vi "frontEnd.vi"(8 "error in (no error)":errorcluster, 11 "ScriptEditorV2 in":refnum<class "ScriptEditorV2.lvclass">) -> (0 "error out":errorcluster, 3 "ScriptEditorV2 out":refnum<class "ScriptEditorV2.lvclass">)   [LabVIEW 2011, in "Views.lvlib" / "ScriptEditor.lvlib" / "ScriptEditorV2.lvclass"]
uses:
  ScriptEditorV2.lvclass
  ScriptEditorV2.lvclass/ScriptEditorV2.ctl
  ScriptEdEvents/ScriptEdEvents.lvclass
  Tools/DatabaseHelpers.lvlib
panel:
  in  "Delete Event":bool
  in  "highlightChannel":bool
  in  "open":bool
  in  "saveAs":bool
  in  "save":bool
  in  "Script Information":string
  out "Multicolumn Listbox":i32[](listbox)
  # "Open"
  # "save"
  # "saveAs"
  # "Highlight"
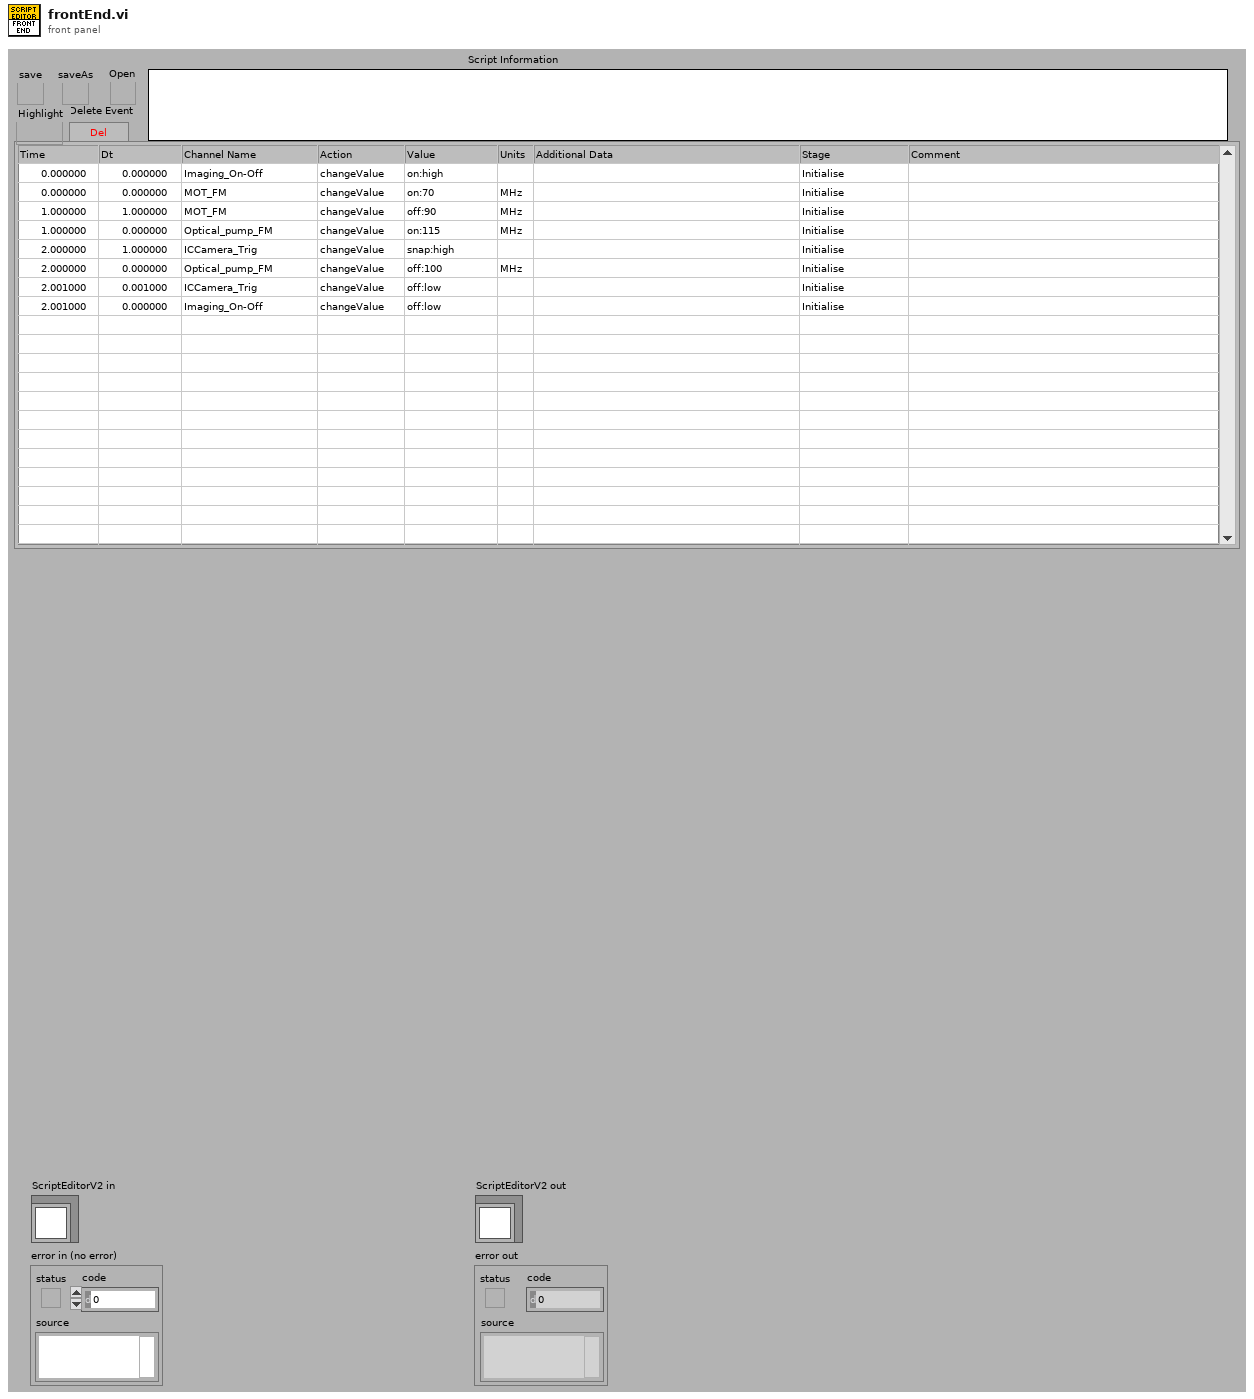
[diagram p1: front panel]
types:
  T1 = typedef "LVPoint32TypeDef.ctl" = cluster{"Horizontal":i32, "Vertical":i32}
  T2 = typedef "LVRowAndColumnTypeDef.ctl" = cluster{"Row":i32, "Column":i32}
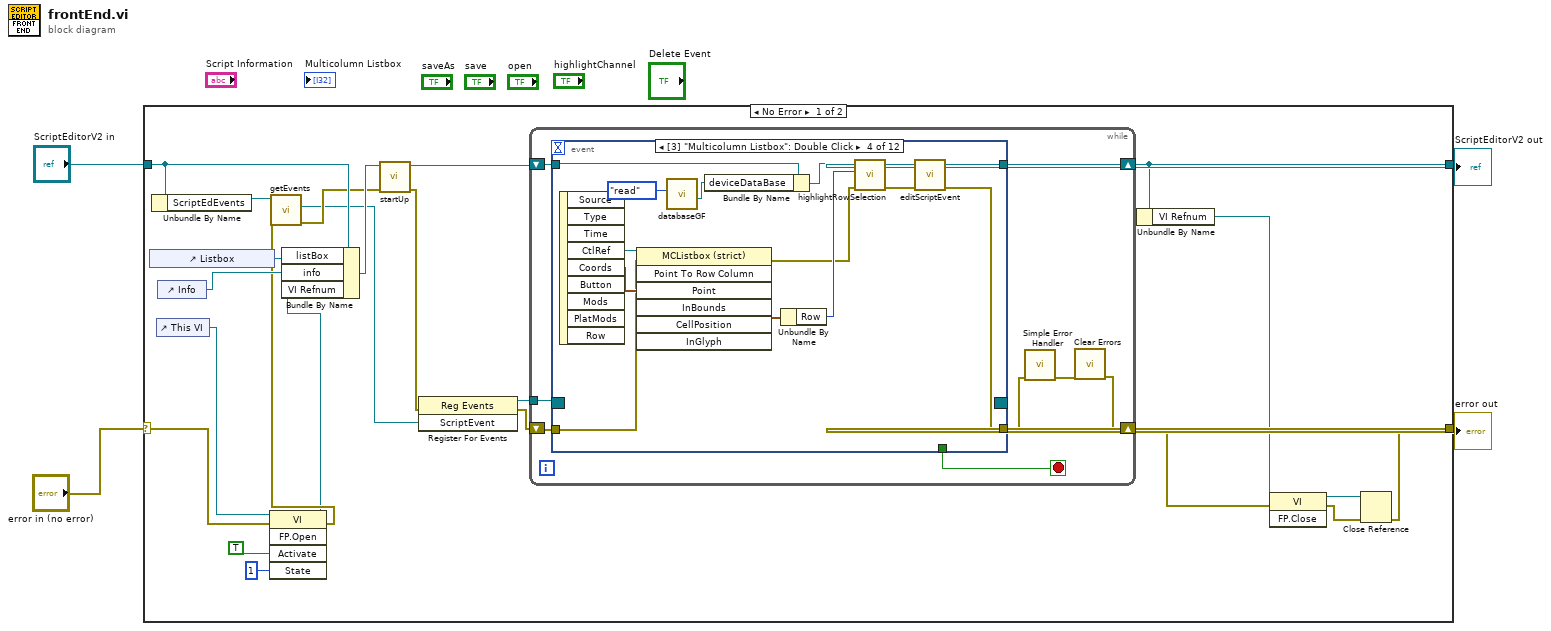
[diagram p0: block diagram]
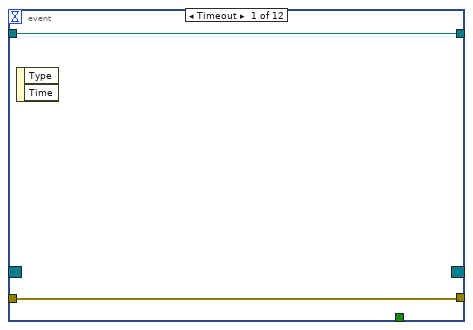
[diagram p2: hidden frame]
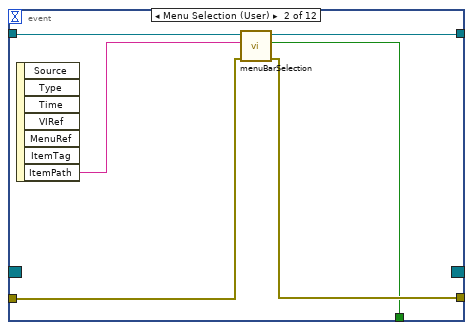
[diagram p3: hidden frame]
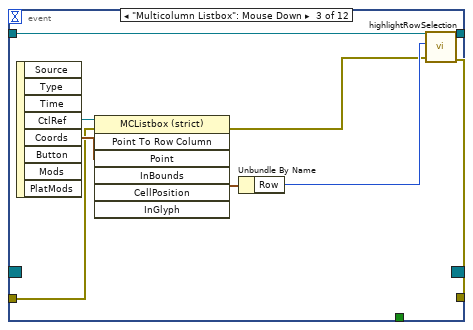
[diagram p4: hidden frame]
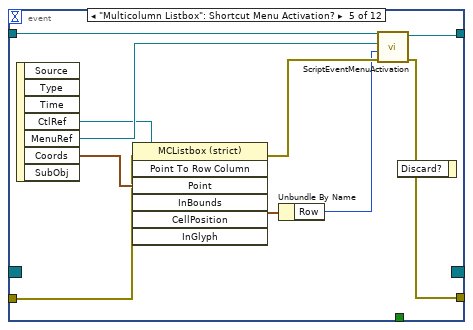
[diagram p5: hidden frame]
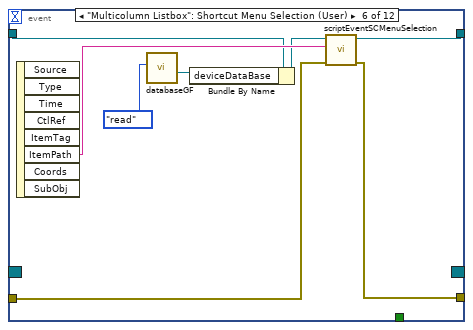
[diagram p6: hidden frame]
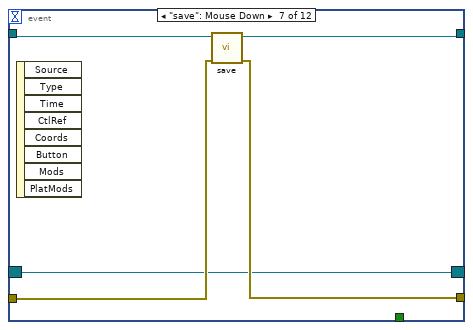
[diagram p7: hidden frame]
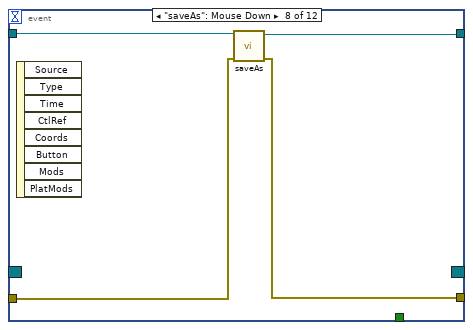
[diagram p8: hidden frame]
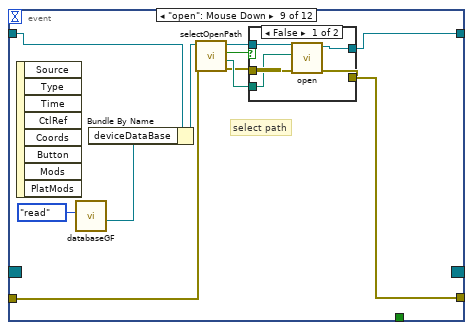
[diagram p9: hidden frame]
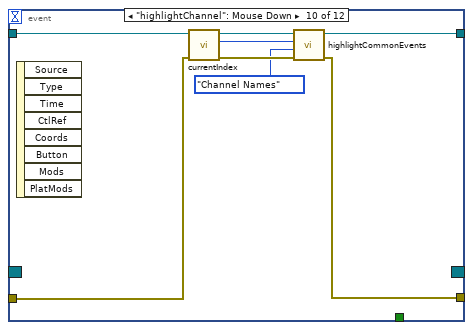
[diagram p11: hidden frame]
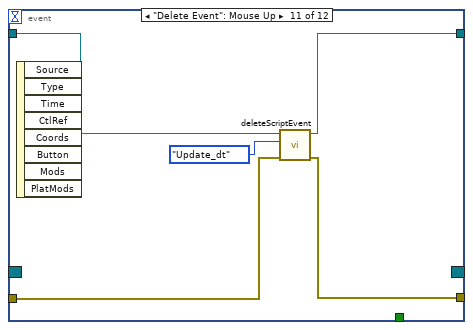
[diagram p12: hidden frame]
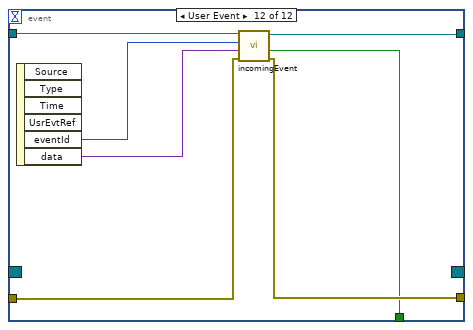
[diagram p13: hidden frame]
diagram:
  n1 = case shown="No Error" "error in (no error)" {
    selector: "error in (no error)" -> [w13 w133]
    tunnel: [w5 w133] -> w3
    tunnel: [w10 w132] -> w1
    tunnel: "ScriptEditorV2 in" -> [w24 w132]
    frame No Error {
      n2 = control-ref of="Listbox"() -> (w17:refnum<vi>)
      n3 = Unbundle By Name(w24) -> ("ScriptEdEvents"=w23:refnum<class "ScriptEdEvents.lvclass">)
      n4 = control-ref of="This VI"() -> (w14:refnum<vi>)
      n5 = control-ref of="Info"() -> (w26:refnum<vi>)
      n6 = invoke class="VI" method="FP.Open"(reference=w14, error in=w13, "Activate"=TRUE, "State"=1) -> (reference out=w11:refnum<vi>, error out=w12:errorcluster)  [unwired: 1 in, 3 out]
      n7 = call-dynamic "getEvents.vi"("error in (no error)"=w12, "ScriptEdEvents in"=w23) -> ("error out"=w21:errorcluster, "ScriptEvent"=w20:refnum<user-event>)  [unwired: 6 in, 2 out]
      n8 = Bundle By Name(cluster=w24, "listBox"=w17, "info"=w26, "VI Refnum"=w11) -> (w25:refnum<class "ScriptEditorV2.lvclass">)
      n9 = call "startUp.vi"("error in (no error)"=w21, "ScriptEditorV2 in"=w25) -> ("error out"=w18:errorcluster, "ScriptEditorV2 out"=w27:refnum<class "ScriptEditorV2.lvclass">)  [unwired: 8 in]
      n10 = register-events(error in=w18, w20) -> (reference out=w22:refnum<event-registration>, error out=w19:errorcluster)  [unwired: 1 in]
      n11 = while {
        shift-right: [w35] -> w10
        shift-left: w27 -> [w31]
        shift-right: [w28] -> w8
        shift-left: w19 -> [w34]
        tunnel: w22 -> [w32]
        stop <- w33 stop-if-true
        n12 = event shown="[3] \"Multicolumn Listbox\": Double Click" {
          selector: w32 -> [_ _ _ _ _ _ w85 _ _ _ _ _]
          dyn-events: [_ _ _ _ _ _ w85 _ _ _ _ _] -> _
          timeout: _ -> [_ _ _ _ _ _ _ _ _ _ _ _]
          tunnel: w31 -> [w37 w43 w45 w54 w76 w79 w89 w93 w96 w115 w121 w131]
          tunnel: [w37 w42 w48 w58 w75 w84 w88 w92 w100 w114 w120 w130] -> w35
          tunnel: [w36 w40 w47 w57 w74 w82 w86 w90 w99 w112 w122 w128] -> w30
          tunnel: w34 -> [w36 w41 w50 w63 w70 w83 w87 w91 w98 w113 w123 w129]
          tunnel: [_ w39 _ _ _ _ _ _ _ _ _ w125] -> w33
          event Timeout {
            n13 = event-data() -> ()  [unwired: 1 in, 2 out]
          }
          event Menu Selection (User) {
            n14 = event-data() -> ("ItemPath"=w38:string)  [unwired: 1 in, 6 out]
            n15 = call "menuBarSelection.vi"("error in (no error)"=w41, "itemPath"=w38, "ScriptEditorV2 in"=w43) -> ("error out"=w40:errorcluster, "close"=w39:bool, "ScriptEditorV2 out"=w42:refnum<class "ScriptEditorV2.lvclass">)  [unwired: 6 in]
          }
          event "Multicolumn Listbox": Mouse Down {
            n16 = event-data() -> ("CtlRef"=w52:refnum<vi>, "Coords"=w51:T1)  [unwired: 1 in, 6 out]
            n17 = invoke class="MCListbox (strict)" method="Point To Row Column"(reference=w52, error in=w50, "Point"=w51) -> (error out=w44:errorcluster, "CellPosition"=w49:T2)  [unwired: 4 in, 5 out]
            n18 = Unbundle By Name(w49) -> ("Row"=w46:i32)
            n19 = call "highlightRowSelection.vi"("error in (no error)"=w44, "rowIndex"=w46, "ScriptEditorV2 in"=w45) -> ("error out"=w47:errorcluster, "ScriptEditorV2 out"=w48:refnum<class "ScriptEditorV2.lvclass">)  [unwired: 7 in]
          }
          event "Multicolumn Listbox": Double Click {
            n20 = event-data() -> ("CtlRef"=w65:refnum<vi>, "Coords"=w64:T1)  [unwired: 1 in, 7 out]
            n21 = invoke class="MCListbox (strict)" method="Point To Row Column"(reference=w65, error in=w63, "Point"=w64) -> (error out=w61:errorcluster, "CellPosition"=w66:T2)  [unwired: 4 in, 5 out]
            n22 = call "databaseGF.vi"("Enum"=enum16{"write", "read"}."read") -> ("deviceDataBase out"=w55:refnum<class "deviceDataBase.lvclass">)  [unwired: 10 in]
            n23 = Bundle By Name(cluster=w54, "deviceDataBase"=w55) -> (w53:refnum<class "ScriptEditorV2.lvclass">)
            n24 = Unbundle By Name(w66) -> ("Row"=w62:i32)
            n25 = call "highlightRowSelection.vi"("error in (no error)"=w61, "rowIndex"=w62, "ScriptEditorV2 in"=w53) -> ("error out"=w59:errorcluster, "ScriptEditorV2 out"=w60:refnum<class "ScriptEditorV2.lvclass">)  [unwired: 7 in]
            n26 = call "editScriptEvent.vi"("error in (no error)"=w59, "ScriptEditorV2 in"=w60) -> ("error out"=w57:errorcluster, "ScriptEditorV2 out"=w58:refnum<class "ScriptEditorV2.lvclass">)  [unwired: 8 in]
          }
          event "Multicolumn Listbox": Shortcut Menu Activation? {
            n27 = event-data() -> ("CtlRef"=w72:refnum<vi>, "MenuRef"=w73:refnum<k9>, "Coords"=w71:T1)  [unwired: 1 in, 4 out]
            n28 = invoke class="MCListbox (strict)" method="Point To Row Column"(reference=w72, error in=w70, "Point"=w71) -> (error out=w68:errorcluster, "CellPosition"=w69:T2)  [unwired: 4 in, 5 out]
            n29 = Unbundle By Name(w69) -> ("Row"=w67:i32)
            n30 = call "ScriptEventMenuActivation.vi"("error in (no error)"=w68, "rowIndex"=w67, "MenuRef"=w73, "ScriptEditorV2 in"=w76) -> ("error out"=w74:errorcluster, "ScriptEditorV2 out"=w75:refnum<class "ScriptEditorV2.lvclass">)  [unwired: 6 in]
            n31 = event-data() -> ()  [unwired: 2 in, 1 out]
          }
          event "Multicolumn Listbox": Shortcut Menu Selection (User) {
            n32 = event-data() -> ("ItemPath"=w81:string)  [unwired: 1 in, 7 out]
            n33 = call "databaseGF.vi"("Enum"=enum16{"write", "read"}."read") -> ("deviceDataBase out"=w77:refnum<class "deviceDataBase.lvclass">)  [unwired: 10 in]
            n34 = Bundle By Name(cluster=w79, "deviceDataBase"=w77) -> (w78:refnum<class "ScriptEditorV2.lvclass">)
            n35 = call "scriptEventSCMenuSelection.vi"("error in (no error)"=w83, "path"=w81, "ScriptEditorV2 in"=w78) -> ("error out"=w82:errorcluster, "ScriptEditorV2 out"=w84:refnum<class "ScriptEditorV2.lvclass">)  [unwired: 7 in]
          }
          event "save": Mouse Down {
            n36 = event-data() -> ()  [unwired: 1 in, 8 out]
            n37 = call "save.vi"("error in (no error)"=w87, "ScriptEditorV2 in"=w89) -> ("error out"=w86:errorcluster, "ScriptEditorV2 out"=w88:refnum<class "ScriptEditorV2.lvclass">)  [unwired: 8 in]
          }
          event "saveAs": Mouse Down {
            n38 = event-data() -> ()  [unwired: 1 in, 8 out]
            n39 = call "saveAs.vi"("error in (no error)"=w91, "ScriptEditorV2 in"=w93) -> ("error out"=w90:errorcluster, "ScriptEditorV2 out"=w92:refnum<class "ScriptEditorV2.lvclass">)  [unwired: 8 in]
          }
          event "open": Mouse Down {
            # "select path"
            n40 = event-data() -> ()  [unwired: 1 in, 8 out]
            n41 = call "databaseGF.vi"("Enum"=enum16{"write", "read"}."read") -> ("deviceDataBase out"=w94:refnum<class "deviceDataBase.lvclass">)  [unwired: 10 in]
            n42 = Bundle By Name(cluster=w96, "deviceDataBase"=w94) -> (w95:refnum<class "ScriptEditorV2.lvclass">)
            n43 = call "selectOpenPath.vi"("error in (no error)"=w98, "ScriptEditorV2 in"=w95) -> ("error out"=w101:errorcluster, "selected path"=w103:path, "notSelected?"=w102:bool, "ScriptEditorV2 out"=w104:refnum<class "ScriptEditorV2.lvclass">)  [unwired: 6 in]
            n44 = case shown="False" w102 {
              tunnel: [w109 w111] -> w100
              tunnel: w101 -> [w108 w110]
              tunnel: [w107 w110] -> w99
              tunnel: w104 -> [w106 w111]
              tunnel: w103 -> [w105 _]
              frame False {
                n45 = call "open.vi"("error in (no error)"=w108, "Path"=w105, "ScriptEditorV2 in"=w106) -> ("error out"=w107:errorcluster, "ScriptEditorV2 out"=w109:refnum<class "ScriptEditorV2.lvclass">)  [unwired: 7 in]
              }
              frame True {
              }
            }
          }
          event "highlightChannel": Mouse Down {
            n46 = event-data() -> ()  [unwired: 1 in, 8 out]
            n47 = call "currentIndex.vi"("error in (no error)"=w113, "ScriptEditorV2 in"=w115) -> ("error out"=w118:errorcluster, "index"=w119:i32, "ScriptEditorV2 out"=w117:refnum<class "ScriptEditorV2.lvclass">)  [unwired: 7 in]
            n48 = call "highlightCommonEvents.vi"("error in (no error)"=w118, "Enum"=enum16{"Channel Names", "Stage"}."Channel Names", "rowIndex"=w119, "ScriptEditorV2 in"=w117) -> ("error out"=w112:errorcluster, "ScriptEditorV2 out"=w114:refnum<class "ScriptEditorV2.lvclass">)  [unwired: 6 in]
          }
          event "Delete Event": Mouse Up {
            n49 = event-data() -> ()  [unwired: 1 in, 8 out]
            n50 = call "deleteScriptEvent.vi"("error in (no error)"=w123, "Enum"=enum16{"Update_dt", "Update_Time"}."Update_dt", "ScriptEditorV2 in"=w121) -> ("error out"=w122:errorcluster, "ScriptEditorV2 out"=w120:refnum<class "ScriptEditorV2.lvclass">)  [unwired: 7 in]
          }
          event User Event {
            n51 = event-data() -> ("eventId"=w127:enum16{"Open", "Save", "Close"}, "data"=w126:variant)  [unwired: 1 in, 4 out]
            n52 = call "incomingEvent.vi"("error in (no error)"=w129, "data"=w126, "eventId"=w127, "ScriptEditorV2 in"=w131) -> ("error out"=w128:errorcluster, "close"=w125:bool, "ScriptEditorV2 out"=w130:refnum<class "ScriptEditorV2.lvclass">)  [unwired: 5 in]
          }
        }
        n53 = call <vilib>:"Simple Error Handler.vi"("error in (no error)"=w30) -> ("error out"=w29:errorcluster)  [unwired: 4 in, 4 out]
        n54 = call <vilib>:"Clear Errors.vi"("error in (no error)"=w29) -> ("error out"=w28:errorcluster)  [unwired: 6 in]
      }
      n55 = Unbundle By Name(w10) -> ("VI Refnum"=w9:refnum<vi>)
      n56 = invoke class="VI" method="FP.Close"(reference=w9, error in=w8) -> (reference out=w6:refnum<vi>, error out=w7:errorcluster)  [unwired: 1 in, 1 out]
      n57 = Close Reference(reference=w6, error in (no error)=w7) -> (error out=w5:errorcluster)
    }
    frame Error {
    }
  }
  "error out" <- w3
  "ScriptEditorV2 out" <- w1
